vi "Error Message Data to XML.vi"(8 "error in (no error)":errorcluster, 10 "Error Message Data":T1, 11 "Error Handler in":refnum<class "XML Log.lvclass">) -> (0 "error out":errorcluster, 3 "Error Handler out":refnum<class "XML Log.lvclass">)   [LabVIEW 2020, in "Error Log Classes.lvlib" / "XML Log.lvclass"]
uses:
  XML Log.lvclass
  Process Classes/Error Handler/Public/TypeDefs/Error Message Data.ctl
  XML Log.lvclass/XML Log.ctl
  <vilib>/xml/Close Reference(NdList).vi
  <vilib>/xml/Close Reference(Node).vi
  <resource>/objmgr/DOMUserDefRef.rc
  <vilib>/xml/NI_XML.lvlib
  Process Classes/Error Handler/Error Handler.lvclass
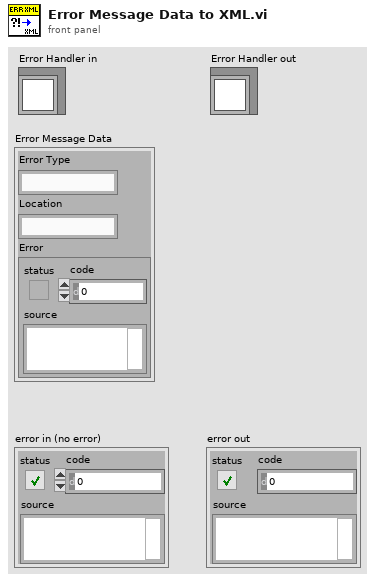
[diagram p1: front panel]
types:
  T1 = typedef "Error Handler.lvclass/Error Message Data.ctl" = cluster{"Error Type":string, "Location":string, "Error":errorcluster}
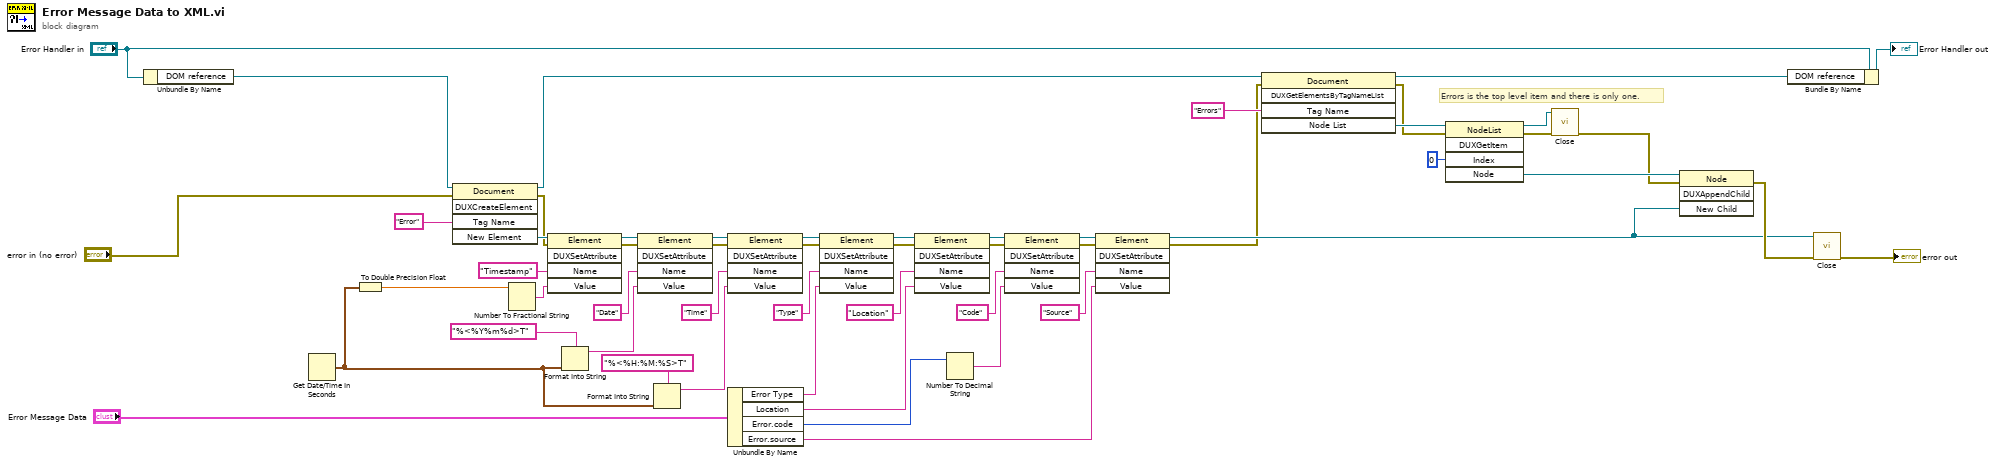
[diagram p0: block diagram]
diagram:
  # "Errors is the top level item and there is only one."
  n1 = Unbundle By Name("Error Handler in") -> ("DOM reference"=w10:refnum<k20>)
  n2 = Get Date/Time In Seconds() -> (seconds since 1Jan1904=w8:timestamp)
  n3 = To Double Precision Float(number=w8) -> (double precision float=w43:dbl)
  n4 = invoke class="Document" method="DUXCreateElement"(reference=w10, error in="error in (no error)", "Tag Name"="Error") -> (reference out=w9:refnum<k20>, error out=w17:errorcluster, "New Element"=w33:refnum<k20>)  [unwired: 2 in, 2 out]
  n5 = Number To Fractional String(number=w43) -> (F-format string=w44:string)  [unwired: 3 in]
  n6 = invoke class="Element" method="DUXSetAttribute"(reference=w33, error in=w17, "Name"="Timestamp", "Value"=w44) -> (reference out=w34:refnum<k20>, error out=w35:errorcluster)  [unwired: 1 in, 3 out]
  n7 = Format Into String(format string="%<%Y%m%d>T", w8) -> (resulting string=w46:string)  [unwired: 2 in, 1 out]
  n8 = invoke class="Element" method="DUXSetAttribute"(reference=w34, error in=w35, "Name"="Date", "Value"=w46) -> (reference out=w37:refnum<k20>, error out=w38:errorcluster)  [unwired: 1 in, 3 out]
  n9 = Format Into String(format string="%<%H:%M:%S>T", w8) -> (resulting string=w48:string)  [unwired: 2 in, 1 out]
  n10 = invoke class="Element" method="DUXSetAttribute"(reference=w37, error in=w38, "Name"="Time", "Value"=w48) -> (reference out=w39:refnum<k20>, error out=w40:errorcluster)  [unwired: 1 in, 3 out]
  n11 = Unbundle By Name("Error Message Data") -> ("Error Type"=w49:string, "Location"=w50:string, "Error.code"=w51:i32, "Error.source"=w53:string)
  n12 = invoke class="Element" method="DUXSetAttribute"(reference=w39, error in=w40, "Name"="Type", "Value"=w49) -> (reference out=w24:refnum<k20>, error out=w25:errorcluster)  [unwired: 1 in, 3 out]
  n13 = invoke class="Element" method="DUXSetAttribute"(reference=w24, error in=w25, "Name"="Location", "Value"=w50) -> (reference out=w26:refnum<k20>, error out=w27:errorcluster)  [unwired: 1 in, 3 out]
  n14 = Number To Decimal String(number=w51) -> (decimal integer string=w52:string)  [unwired: 1 in]
  n15 = invoke class="Element" method="DUXSetAttribute"(reference=w26, error in=w27, "Name"="Code", "Value"=w52) -> (reference out=w28:refnum<k20>, error out=w29:errorcluster)  [unwired: 1 in, 3 out]
  n16 = invoke class="Element" method="DUXSetAttribute"(reference=w28, error in=w29, "Name"="Source", "Value"=w53) -> (reference out=w14:refnum<k20>, error out=w7:errorcluster)  [unwired: 1 in, 3 out]
  n17 = invoke class="Document" method="DUXGetElementsByTagNameList"(reference=w9, error in=w7, "Tag Name"="Errors") -> (reference out=w11:refnum<k20>, error out=w4:errorcluster, "Node List"=w5:refnum<k20>)  [unwired: 2 in, 2 out]
  n18 = invoke class="NodeList" method="DUXGetItem"(reference=w5, error in=w4, "Index"=0) -> (reference out=w2:refnum<k20>, error out=w3:errorcluster, "Node"=w12:refnum<k20>)  [unwired: 2 in, 2 out]
  n19 = call-poly <vilib>:"Close.vi"("error in (no error)"=w3, "node list"=w2) -> ("error out"=w6:errorcluster)  [unwired: 7 in]
  n20 = invoke class="Node" method="DUXAppendChild"(reference=w12, error in=w6, "New Child"=w14) -> (error out=w16:errorcluster)  [unwired: 1 in, 3 out]
  n21 = Bundle By Name(cluster="Error Handler in", "DOM reference"=w11) -> (→"Error Handler out":refnum<class "XML Log.lvclass">)
  n22 = call-poly <vilib>:"Close.vi"("error in (no error)"=w16, "node"=w14) -> ("error out"=→"error out":errorcluster)  [unwired: 7 in]
